vi "initialize.vi"(0 "HGF_DIMCommand":refnum<class "HGF_DIMCommand.lvclass">, 3 "initializationData":variant, 5 "error in (no error)":errorcluster, 7 "binaryString":string, 8 "I8 Array":i8[](array[numeric]), 9 "prependSize? (T)":bool, 11 "byteOrder (0:big-endian, network order)":T1(ring)) -> (14 "dup HGF_DIMCommand":refnum<class "HGF_DIMCommand.lvclass">, 17 "found?":bool, 19 "error out":errorcluster)   [LabVIEW 2012, in "HGF_DIM.lvlib" / "HGF_DIMCommand.lvclass"]
doc: "This is a dynamic dispatch VI to be implemented by child classes to initialize their attributes.\n\n<B>Recommendation:</B> Use Variant for initialization data."
uses:
  HGF_DIMCommand.lvclass
  HGF_BaseClasses/HGF_PVSubscriber/HGF_PVSubscriber.lvclass
  HGF_DIMCommand.lvclass/HGF_DIMCommand.ctl
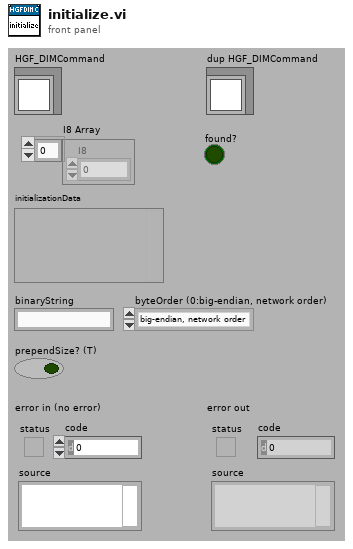
[diagram p1: front panel]
types:
  T1 = enum16{"big-endian, network order", "native, host order", "little-endian"}
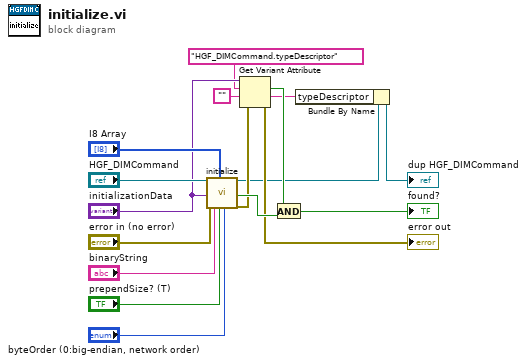
[diagram p0: block diagram]
diagram:
  n1 = call-parent "initialize.vi"("HGV_PVBase"="HGF_DIMCommand", "initializationData"="initializationData", "error in (no error)"="error in (no error)", "binaryString"="binaryString", "I8 Array"="I8 Array", "prependSize? (T)"="prependSize? (T)", "byteOrder (0:big-endian, network order)"="byteOrder (0:big-endian, network order)") -> ("HGV_PVBase"=w3:refnum<class "HGF_DIMCommand.lvclass">, "found?"=w7:bool, "error out"=w5:errorcluster)  [unwired: 10 out]
  n2 = Get Variant Attribute(Variant="initializationData", name="HGF_DIMCommand.typeDescriptor", default value (empty Variant)="", error in=w5) -> (found=w8:bool, value=w1:string, error out=→"error out":errorcluster)  [unwired: 1 out]
  n3 = And(x=w8, y=w7) -> (x .and. y?=→"found?":bool)
  n4 = Bundle By Name(cluster=w3, "typeDescriptor"=w1) -> (→"dup HGF_DIMCommand":refnum<class "HGF_DIMCommand.lvclass">)
